vi "SBML_Compartments_Def.vi"(8 "error in (no error)":errorcluster, 11 "Input SBML File":string) -> (0 "error out":errorcluster, 2 "Compartments Definition":string[][](table), 3 "Compartments_Cnt":i32)   [LabVIEW 2014]
doc: "This VI extract the information of species present in SBML file. It takes the complete SBML file as input, and outputs: \nSp_Cnt --> How many species are there\nS_Id_Arr --> Array of species\nSp_Name --> Array containing the name of species\nSp_Init_Amnt --> Array containing the initial amount of species\n\nDesigned by HB\nhaba@dtu.dk"
panel:
  out "Constant":string[](array[string])
  out "Unit":string[](array[string])
  out "Size":string[](array[string])
  out "Spatial Dimensions":string[](array[string])
  out "Comp_Name":string[](array[string])
  out "Comp_ID":string[](array[string])
  out "List of Units":string
  # "Names"
  # "Initial Amount"
  # "ID"
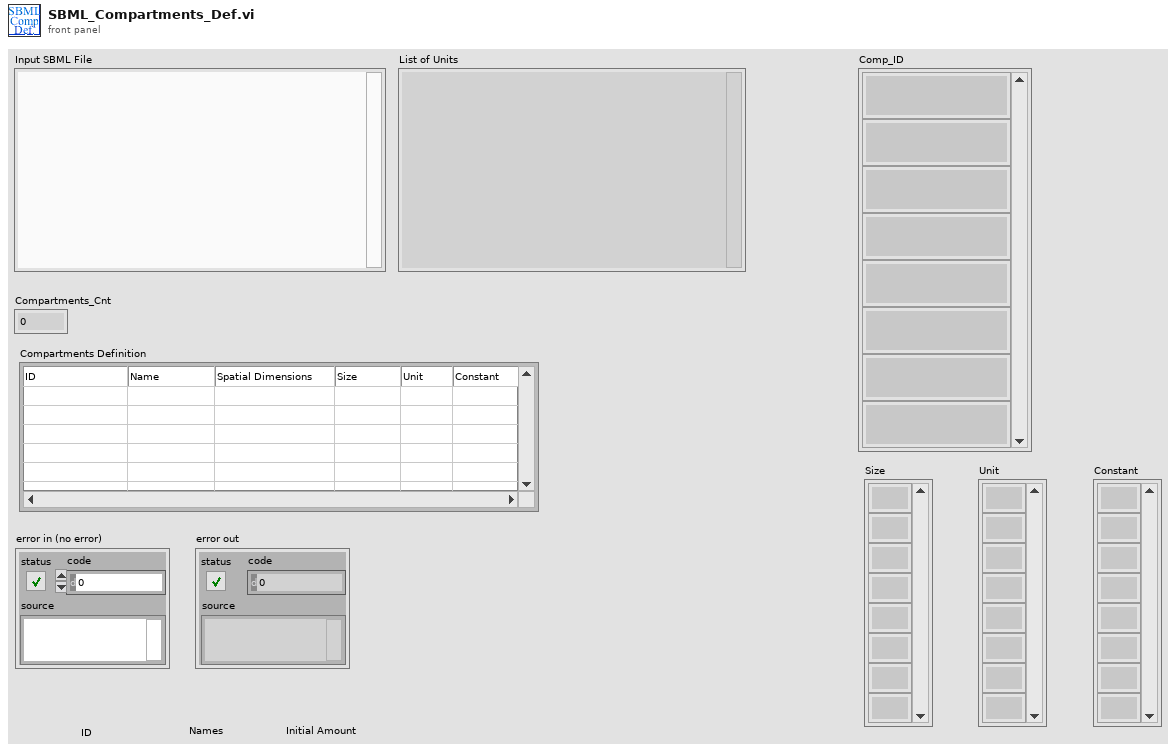
[diagram p1: front panel]
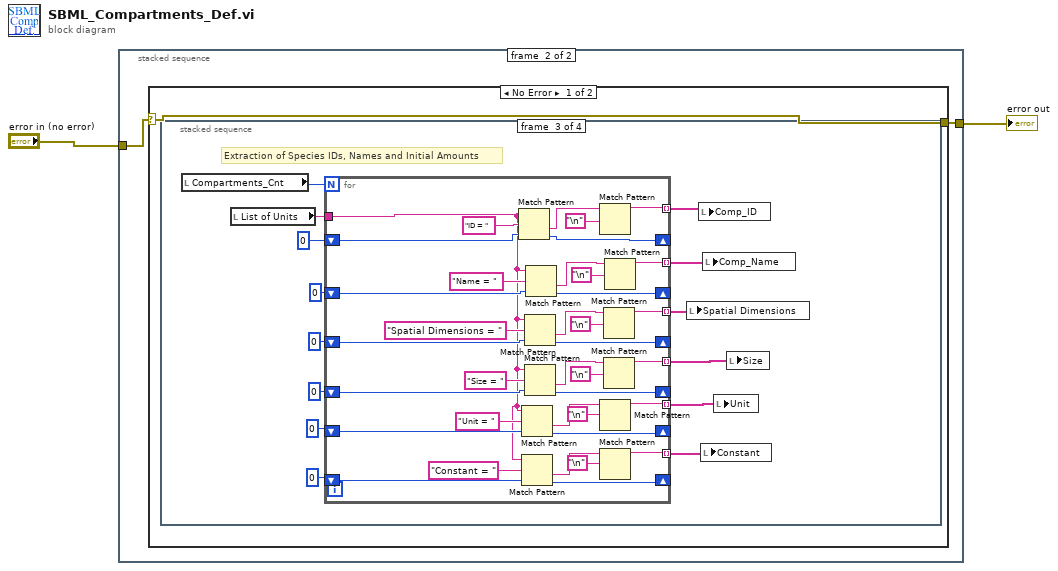
[diagram p0: block diagram]
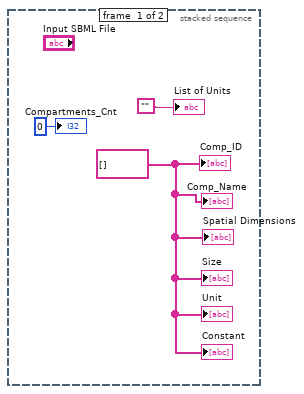
[diagram p2: hidden frame]
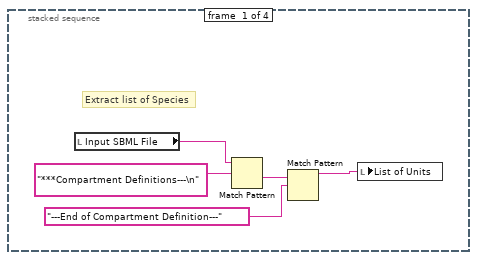
[diagram p3: hidden frame]
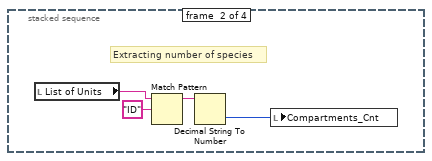
[diagram p4: hidden frame]
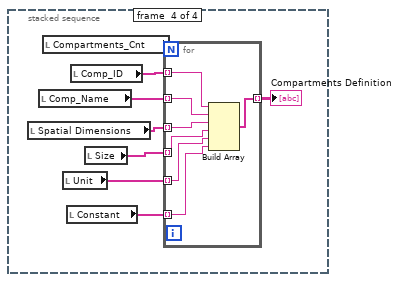
[diagram p5: hidden frame]
diagram:
  n1 = stacked-sequence {
    tunnel: "error in (no error)" -> [_ w6]
    tunnel: [_ w7] -> w1
    frame #0 {
      w3 = string[] [] ("Sp_Id_Arr")
      "List of Units" <- "" ("Full SBML File")
      "Compartments_Cnt" <- 0 ("Sp_cnt")
      "Comp_ID" <- w3
      "Comp_Name" <- w3
      "Spatial Dimensions" <- w3
      "Size" <- w3
      "Unit" <- w3
      "Constant" <- w3
    }
    frame #1 {
      n2 = case shown="No Error" w6 {
        selector: w6 -> [w8 w84]
        tunnel: [w8 w84] -> w7
        frame No Error {
          n3 = stacked-sequence {
            frame #0 {
              # "Extract list of Species"
              n4 = local read "Input SBML File"() -> (w10:string)
              n5 = Match Pattern(string=w10, regular expression="***Compartment Definitions---\n") -> (after substring=w12:string)  [unwired: 1 in, 3 out]
              n6 = Match Pattern(string=w12, regular expression="---End of Compartment Definition---") -> (before substring=w9:string)  [unwired: 1 in, 3 out]
              n7 = local write "List of Units"(w9) -> ()
            }
            frame #1 {
              # "Extracting number of species"
              n8 = local read "List of Units"() -> (w14:string)
              n9 = Match Pattern(string=w14, regular expression="ID") -> (before substring=w16:string)  [unwired: 1 in, 3 out]
              n10 = Decimal String To Number(string=w16) -> (number=w15:i32)  [unwired: 2 in, 1 out]
              n11 = local write "Compartments_Cnt"(w15) -> ()
            }
            frame #2 {
              # "Extraction of Species IDs, Names and Initial Amounts"
              n12 = local read "Compartments_Cnt"() -> (w28:i32)
              n13 = local read "List of Units"() -> (w29:string)
              n14 = for {
                N: w28 -> [_]
                tunnel: w29 -> [w32]
                shift-right: [w65] -> _
                shift-left: 0 ("offset past match") -> [w64]
                shift-right: [w60] -> _
                shift-left: 0 ("offset past match") -> [w59]
                tunnel: [w58] -> w27 mode=indexing
                tunnel: [w57] -> w26 mode=indexing
                shift-right: [w55] -> _
                shift-left: 0 ("offset of match") -> [w56]
                tunnel: [w54] -> w24 mode=indexing
                shift-right: [w48] -> _
                shift-left: 0 ("offset past match") -> [w49]
                tunnel: [w50] -> w23 mode=indexing
                shift-right: [w42] -> _
                shift-left: 0 ("offset past match") -> [w43]
                tunnel: [w44] -> w21 mode=indexing
                shift-right: [w34] -> _
                shift-left: 0 ("offset of match") -> [w33]
                tunnel: [w35] -> w19 mode=indexing
                n15 = Match Pattern(string=w32, regular expression="ID = ", offset (0)=w59) -> (after substring=w61:string, offset past match=w60:i32)  [unwired: 2 out]
                n16 = Match Pattern(string=w32, regular expression="Unit = ", offset (0)=w56) -> (after substring=w53:string, offset past match=w55:i32)  [unwired: 2 out]
                n17 = Match Pattern(string=w32, regular expression="Constant = ", offset (0)=w33) -> (after substring=w36:string, offset past match=w34:i32)  [unwired: 2 out]
                n18 = Match Pattern(string=w32, regular expression="Spatial Dimensions = ", offset (0)=w64) -> (after substring=w68:string, offset past match=w65:i32)  [unwired: 2 out]
                n19 = Match Pattern(string=w32, regular expression="Size = ", offset (0)=w43) -> (after substring=w39:string, offset past match=w42:i32)  [unwired: 2 out]
                n20 = Match Pattern(string=w32, regular expression="Name = ", offset (0)=w49) -> (after substring=w45:string, offset past match=w48:i32)  [unwired: 2 out]
                n21 = Match Pattern(string=w61, regular expression="\n") -> (before substring=w57:string)  [unwired: 1 in, 3 out]
                n22 = Match Pattern(string=w53, regular expression="\n") -> (before substring=w54:string)  [unwired: 1 in, 3 out]
                n23 = Match Pattern(string=w36, regular expression="\n") -> (before substring=w35:string)  [unwired: 1 in, 3 out]
                n24 = Match Pattern(string=w68, regular expression="\n") -> (before substring=w58:string)  [unwired: 1 in, 3 out]
                n25 = Match Pattern(string=w39, regular expression="\n") -> (before substring=w44:string)  [unwired: 1 in, 3 out]
                n26 = Match Pattern(string=w45, regular expression="\n") -> (before substring=w50:string)  [unwired: 1 in, 3 out]
              }
              n27 = local write "Spatial Dimensions"(w27) -> ()
              n28 = local write "Comp_ID"(w26) -> ()
              n29 = local write "Constant"(w19) -> ()
              n30 = local write "Comp_Name"(w23) -> ()
              n31 = local write "Unit"(w24) -> ()
              n32 = local write "Size"(w21) -> ()
            }
            frame #3 {
              n33 = local read "Spatial Dimensions"() -> (w73:string[])
              n34 = local read "Comp_Name"() -> (w75:string[])
              n35 = local read "Compartments_Cnt"() -> (w74:i32)
              n36 = local read "Unit"() -> (w70:string[])
              n37 = local read "Constant"() -> (w69:string[])
              n38 = local read "Comp_ID"() -> (w76:string[])
              n39 = local read "Size"() -> (w71:string[])
              n40 = for {
                N: w74 -> [_]
                tunnel: w76 -> [w83] mode=indexing
                tunnel: w75 -> [w82] mode=indexing
                tunnel: [w81] -> w72 mode=indexing
                tunnel: w73 -> [w80] mode=indexing
                tunnel: w71 -> [w79] mode=indexing
                tunnel: w70 -> [w78] mode=indexing
                tunnel: w69 -> [w77] mode=indexing
                n41 = Build Array(w83, w82, w80, w79, w78, w77) -> (w81:string[])
              }
              "Compartments Definition" <- w72
            }
          }
        }
        frame Error {
        }
      }
    }
  }
  "error out" <- w1
